vi "PH_SHS_Analysis_Statistician.Pack Dataset.vi"(0 "i ref in":refnum<vi>, 5 "error in":errorcluster) -> (14 "i ref out":refnum<vi>, 15 "Dataset Legend":string[](array[string]), 16 "Dataset chosen?":bool[](array[boolean]), 17 "Timebase":dbl[](array[numeric]), 18 "Dataset":dbl[][](array[numeric]), 19 "error out":errorcluster)   [LabVIEW 2014, in "PH_SHS_Analysis_Statistician.lvlib"]
doc: "This VI creates the dataset (Timebase, Data) out of the stored data."
uses:
  PH_SHS_Analysis_Statistician.lvlib
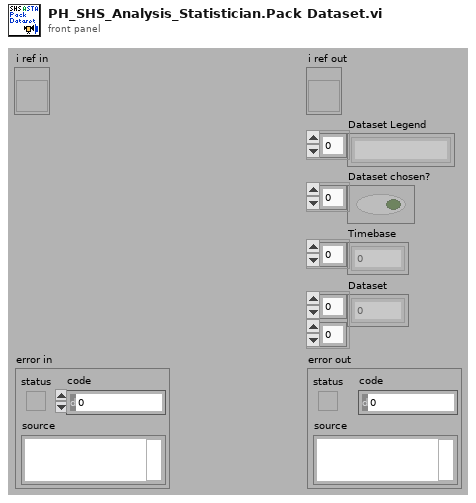
[diagram p1: front panel]
types:
  T1 = typedef "PH_SHS_Analysis_Statistician.lvlib/PH_SHS_Analysis_Statistician.i attribute.ctl" = cluster{"GUI Refs ":cluster{"Status":refnum<vi>, "Result Graph":refnum<vi>, "Mean Data 1":refnum<vi>, "Std Dev Data 1":refnum<vi>, "Mean Data 2":refnum<vi>, "Std Dev Data 2":refnum<vi>, "Mean Data 3":refnum<vi>, "Std Dev Data 3":refnum<vi>, "Dummy Mean":refnum<vi>, "Dummy Std Dev":refnum<vi>, "Export Data":refnum<vi>, "Data 1":refnum<vi>, "Data 2":refnum<vi>, "Data 3":refnum<vi>, "Stat or Trend":refnum<vi>, "Delete":refnum<vi>, "Analyzer":refnum<vi>, "Current Zernike Coefficients":refnum<vi>, "PtV [Lambda]":refnum<vi>, "sample length":refnum<vi>}, "Analyzer":string, "Stat or Trend":bool, "Data 1":i16, "Data 2":i16, "Data 3":i16, "Data":T2[], "sample length":i32, "Datasets strored":i32, "Dataarray Size":i32}
  T2 = typedef "PH_SHS_Analysis.lvlib/PH_SHS_Analysis.Zernike Dataset.ctl" = cluster{"State":T3, "Time Stamp":timestamp, "PtV [lambda]":dbl, "Zernicke Coefficients":T4}
  T3 = typedef "PH_StatusHandler.lvlib/PH_StatusHandler.Status.ctl" = i16
  T4 = typedef "PH_SHS_Analysis.lvlib/PH_SHS_Analysis.Zernike Coefficients.ctl" = cluster{"Tilt x":dbl, "Tilt y":dbl, "Defocus":dbl, "Astig 0°":dbl, "Astig 45°":dbl, "Coma x":dbl, "Coma y":dbl, "Spherical":dbl, "Trefoil 0°":dbl, "Trefoil 30°":dbl, "2nd Astig 0°":dbl, "2nd Astig 45°":dbl, "2nd Coma x":dbl, "2nd Coma y":dbl, "2nd Spherical":dbl}
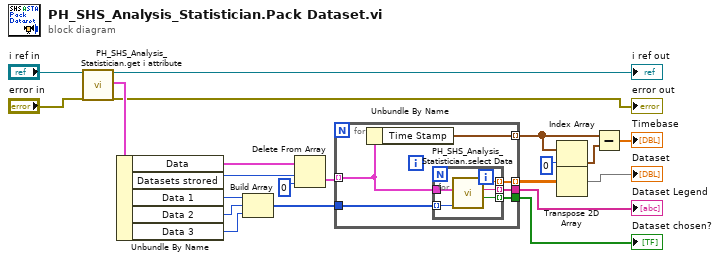
[diagram p0: block diagram]
diagram:
  n1 = call "PH_SHS_Analysis_Statistician.get i attribute.vi"("i ref in"="i ref in", "error in (no error)"="error in") -> ("i ref out"=→"i ref out":refnum<vi>, "i attribute"=w18:T1, "error out"=→"error out":errorcluster)  [unwired: 15 in]
  n2 = Unbundle By Name(w18) -> ("Data"=w4:T2[], "Datasets strored"=w2:i32, "Data 1"=w19:i16, "Data 2"=w20:i16, "Data 3"=w21:i16)
  n3 = Build Array(w19, w20, w21) -> (w7:i16[])
  n4 = Delete From Array(array=w4, length=w2, index=0) -> (deleted portion=w3:T2[])  [unwired: 1 out]
  n5 = for {
    tunnel: w3 -> [w27] mode=indexing
    tunnel: [w22] -> w8 mode=indexing
    tunnel: [w26] -> w10
    tunnel: [w25] -> w13
    tunnel: [w24] -> w9 mode=indexing
    tunnel: w7 -> [w23]
    n6 = Unbundle By Name(w27) -> ("Time Stamp"=w22:timestamp)
    n7 = for {
      tunnel: w27 -> [w29]
      tunnel: [w32] -> w26 mode=indexing
      tunnel: [w31] -> w25 mode=indexing
      tunnel: [w30] -> w24 mode=indexing
      tunnel: w23 -> [w28] mode=indexing
      n8 = call "PH_SHS_Analysis_Statistician.select Data.vi"("Data Selector"=w28, "SHS Analyzer Dataset"=w29) -> ("Data chosen?"=w31:bool, "Data Legend"=w32:string, "Data"=w30:dbl)  [unwired: 5 in]
    }
  }
  "Dataset chosen?" <- w13
  "Dataset Legend" <- w10
  n9 = Index Array(array=w8, index=0) -> (element=w5:timestamp)
  n10 = Transpose 2D Array(2D array=w9) -> (transposed array=→"Dataset":dbl[][])
  n11 = Subtract(x=w8, y=w5) -> (x-y=→"Timebase":dbl[])
